vi "YKMW100 Determine Power Relay Status.vi"(8 "Error In":errorcluster, 10 "Module Number":i32, 11 "Full Module List":string[](array[string])) -> (0 "Error Out":errorcluster, 1 "Intellifaucet Status (0=On and 1=Off)":i32, 2 "DO Card Detected for Module 5":bool, 3 "Relay Status (0=On and 1=Off)":i32)   [LabVIEW 2016]
uses:
  <vilib>/Utility/error.llb/whitespace.ctl
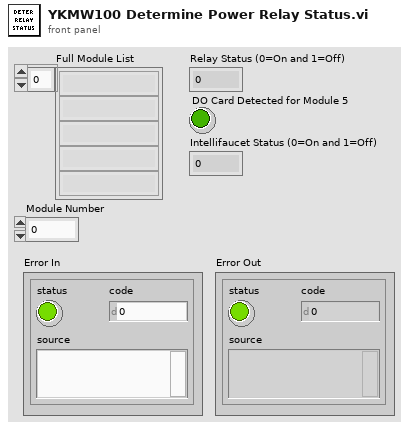
[diagram p1: front panel]
types:
  T1 = typedef "whitespace.ctl" = u16
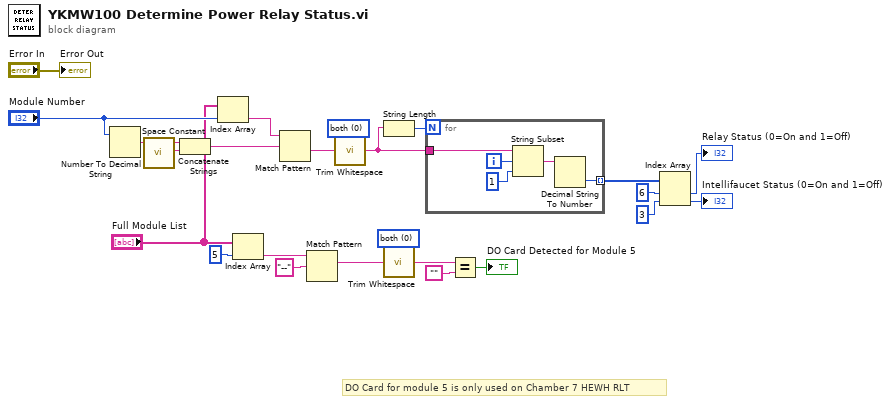
[diagram p0: block diagram]
diagram:
  w8 = T1 0 items=["both", "start of string", "end of string"] ("location (both)")
  w15 = T1 0 items=["both", "start of string", "end of string"] ("location (both)")
  # "DO Card for module 5 is only used on Chamber 7 HEWH RLT"
  n1 = Number To Decimal String(number="Module Number") -> (decimal integer string=w22:string)  [unwired: 1 in]
  n2 = call <vilib>:"Space Constant.vi"() -> ("String"=w23:string)
  n3 = Concatenate Strings(w22, w23) -> (w24:string)
  n4 = Index Array(array="Full Module List", index="Module Number") -> (element=w13:string)
  n5 = Index Array(array="Full Module List", index=5) -> (element=w6:string)
  n6 = Match Pattern(string=w13, regular expression=w24) -> (after substring=w14:string)  [unwired: 1 in, 3 out]
  n7 = Match Pattern(string=w6, regular expression="--") -> (match substring=w10:string)  [unwired: 1 in, 3 out]
  n8 = call <vilib>:"Trim Whitespace.vi"("string"=w14, "location (both)"=w15) -> ("trimmed string"=w17:string)
  n9 = String Length(string=w17) -> (length=w16:i32)
  n10 = call <vilib>:"Trim Whitespace.vi"("string"=w10, "location (both)"=w8) -> ("trimmed string"=w12:string)
  n11 = for {
    N: w16 -> [_]
    tunnel: w17 -> [w28]
    tunnel: [w25] -> w18 mode=indexing
    i -> [w27]
    n12 = String Subset(string=w28, offset (0)=w27, length (rest)=1 ("length (rest)")) -> (substring=w26:string)
    n13 = Decimal String To Number(string=w26) -> (number=w25:i32)  [unwired: 2 in, 1 out]
  }
  n14 = Equal?(x=w12, y="") -> (x = y?=→"DO Card Detected for Module 5":bool)
  n15 = Index Array(array=w18, index #1=6 ("index"), index #2=3 ("index")) -> (element #1=→"Relay Status (0=On and 1=Off)":i32, element #2=→"Intellifaucet Status (0=On and 1=Off)":i32)
  "Error Out" <- "Error In"
